vi "Pre Launch Init.vi"(11 "WebSocket Service Actor in":refnum<class "WebSocket Service Actor.lvclass">) -> (0 "error out":errorcluster, 3 "WebSocket Service Actor out":refnum<class "WebSocket Service Actor.lvclass">)   [LabVIEW 2016, in "WebSocket Actor.lvlib" / "WebSocket Service Actor.lvclass"]
doc: "(<B>Filename</B>: Actor Framework.lvlib:Actor.lvclass:Pre Launch Init.vi)\n\nDefines behavior that occurs after the Launch Nested Actor method is invoked but before the actor's Actor Core method begins running.\n\nBy default, this method does nothing. A descendant class may override it to define behavior."
uses:
  WebSocket Service Actor.lvclass
  <vilib>/ActorFramework/Actor/Actor.lvclass
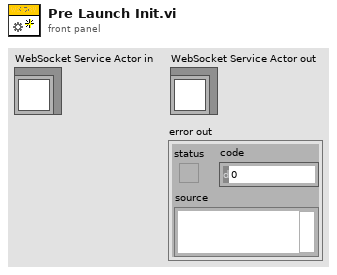
[diagram p1: front panel]
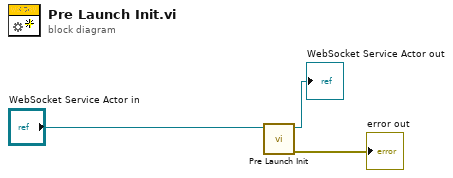
[diagram p0: block diagram]
diagram:
  n1 = call-parent "Pre Launch Init.vi"("Actor in"="WebSocket Service Actor in") -> ("error out"=→"error out":errorcluster, "Actor out"=→"WebSocket Service Actor out":refnum<class "WebSocket Service Actor.lvclass">)  [unwired: 9 in]
